vi "gfitsio-write-key-logical.vi"(6 "comment":string, 7 "keyname":string, 8 "error in (no error)":errorcluster, 9 "value":bool, 11 "gfits refnum":T1) -> (0 "error out":errorcluster, 3 "dup gfits refnum":T1)   [LabVIEW 2023, in "gfitsio.lvlib"]
doc: "Write a keyword of the appropriate data type into the current HDU. If the keyword already exists it will be overwritten. Otherwise a new keyword will be appended to the header."
uses:
  gfitsio.lvlib
  cfitsio-datatypes.ctl
  gfitsio.dll
  gfitsio-refnum.ctl
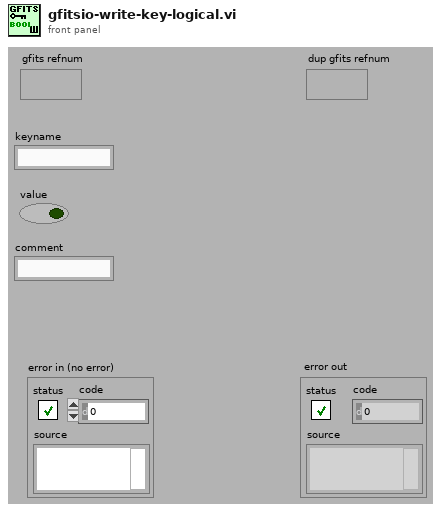
[diagram p1: front panel]
types:
  T1 = typedef "gfitsio.lvlib/gfitsio-refnum.ctl" = refnum<k1>
  T2 = typedef "gfitsio.lvlib/cfitsio-datatypes.ctl" = i32
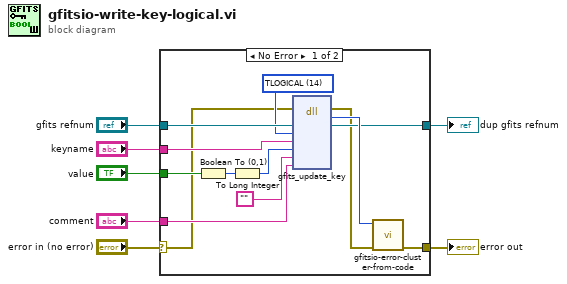
[diagram p0: block diagram]
diagram:
  n1 = case shown="No Error" "error in (no error)" {
    selector: "error in (no error)" -> [w9 w22]
    tunnel: [w19 w22] -> w3
    tunnel: "gfits refnum" -> [w17 w21]
    tunnel: [w18 w21] -> w1
    tunnel: "keyname" -> [w15 _]
    tunnel: "value" -> [w14 _]
    tunnel: "comment" -> [w13 _]
    frame No Error {
      w16 = T2 14 items=["TBIT"=1, "TBYTE  (U8)"=11, "TSBYTE  (I8)"=12, "TLOGICAL"=14, "TSTRING"=16, "TUSHORT  (U16)"=20, "TSHORT  (I16)"=21, "TUINT"=31, "TULONG  (U32)"=40, "TLONG  (I32)"=41, "TFLOAT  (SGL)"=42, "TLONGLONG  (I64)"=81, "TDOUBLE  (DBL)"=82, "TCOMPLEX  (CSG)"=83, "TDOUBLECOMPLEX  (CDB)"=163] ("cfitsio datatype")
      n2 = Boolean To (0,1)(Boolean=w14) -> (0, 1=w11:i16)
      n3 = To Long Integer(number=w11) -> (32bit integer=w10:i32)
      n4 = dll-call lib="gfitsio.dll" fn="gfits_update_key"(error in=w9, "refnum"=w17, "datatype"=w16, "keyname"=w15, "value"=w10, "unit"="", "comment"=w13) -> (error out=w8:errorcluster, "return type"=w20:i32, "refnum"=w18:T1)  [unwired: 6 in, 2 out]
      n5 = call "gfitsio-error-cluster-from-code.vi"("error in (no error)"=w8, "error code"=w20) -> ("error out"=w19:errorcluster)  [unwired: 9 out]
    }
    frame Error {
    }
  }
  "error out" <- w3
  "dup gfits refnum" <- w1
